vi "Get CSV Row.vi"(8 "error in (no error)":errorcluster, 11 "Trace in":refnum<class "Trace.lvclass">) -> (0 "error out":errorcluster, 2 "CSV Row":string, 3 "Trace out":refnum<class "Trace.lvclass">)   [LabVIEW 2014, in "Robot Actor Framework.lvlib" / "Trace.lvlib" / "Trace.lvclass"]
uses:
  Trace.lvclass
  Trace.lvclass/Trace.ctl
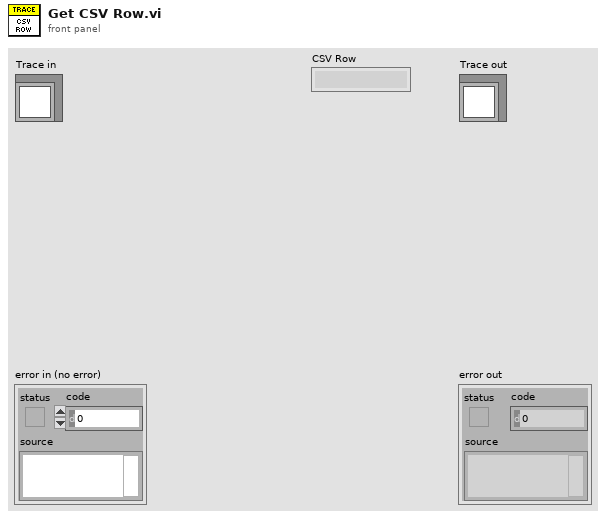
[diagram p1: front panel]
types:
  T1 = enum16{"Critical", "Error", "Warning", "Informational", "Debug"}
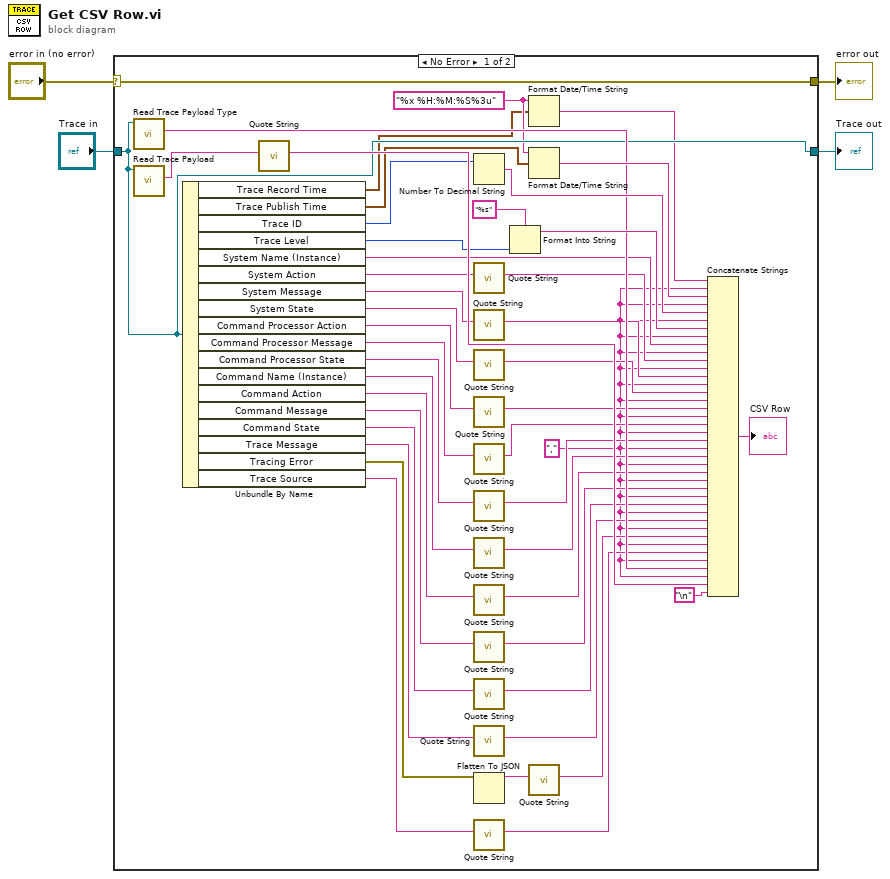
[diagram p0: block diagram]
diagram:
  n1 = case shown="No Error" "error in (no error)" {
    selector: "error in (no error)" -> [w50 w52]
    tunnel: [w50 w52] -> w3
    tunnel: [w33 w51] -> w1
    tunnel: "Trace in" -> [w33 w51]
    frame No Error {
      w8 = "%x %H:%M:%S%3u" ("time format string (%c)")
      w5 = "," ("string")
      n2 = call-dynamic "Read Trace Payload Type.vi"("Trace in"=w33) -> ("Trace Payload Type"=w41:string)  [unwired: 8 in, 2 out]
      n3 = call-dynamic "Read Trace Payload.vi"("Trace in"=w33) -> ("Trace Payload"=w44:string)  [unwired: 8 in, 2 out]
      n4 = Unbundle By Name(w33) -> ("Trace Record Time"=w7:timestamp, "Trace Publish Time"=w36:timestamp, "Trace ID"=w37:u32, "Trace Level"=w38:T1, "System Name (Instance)"=w39:string, "System Action"=w40:string, "System Message"=w20:string, "System State"=w32:string, "Command Processor Action"=w35:string, "Command Processor Message"=w18:string, "Command Processor State"=w29:string, "Command Name (Instance)"=w24:string, "Command Action"=w26:string, "Command Message"=w19:string, "Command State"=w22:string, "Trace Message"=w28:string, "Tracing Error"=w15:errorcluster, "Trace Source"=w12:string)
      n5 = call "Quote String.vi"("String In"=w44) -> ("Quoted String"=w43:string)  [unwired: 10 in]
      n6 = Number To Decimal String(number=w37) -> (decimal integer string=w49:string)  [unwired: 1 in]
      n7 = call "Quote String.vi"("String In"=w40) -> ("Quoted String"=w10:string)  [unwired: 10 in]
      n8 = call "Quote String.vi"("String In"=w20) -> ("Quoted String"=w9:string)  [unwired: 10 in]
      n9 = call "Quote String.vi"("String In"=w32) -> ("Quoted String"=w31:string)  [unwired: 10 in]
      n10 = call "Quote String.vi"("String In"=w35) -> ("Quoted String"=w34:string)  [unwired: 10 in]
      n11 = call "Quote String.vi"("String In"=w18) -> ("Quoted String"=w17:string)  [unwired: 10 in]
      n12 = call "Quote String.vi"("String In"=w29) -> ("Quoted String"=w30:string)  [unwired: 10 in]
      n13 = call "Quote String.vi"("String In"=w24) -> ("Quoted String"=w23:string)  [unwired: 10 in]
      n14 = call "Quote String.vi"("String In"=w26) -> ("Quoted String"=w25:string)  [unwired: 10 in]
      n15 = call "Quote String.vi"("String In"=w19) -> ("Quoted String"=w16:string)  [unwired: 10 in]
      n16 = call "Quote String.vi"("String In"=w22) -> ("Quoted String"=w21:string)  [unwired: 10 in]
      n17 = call "Quote String.vi"("String In"=w28) -> ("Quoted String"=w27:string)  [unwired: 10 in]
      n18 = Flatten To JSON(anything=w15) -> (JSON string=w14:string)  [unwired: 2 in, 1 out]
      n19 = call "Quote String.vi"("String In"=w12) -> ("Quoted String"=w11:string)  [unwired: 10 in]
      n20 = Format Into String(format string="%s", w38) -> (resulting string=w47:string)  [unwired: 2 in, 1 out]
      n21 = Format Date/Time String(time format string (%c)=w8, seconds (now)=w7) -> (date/time string=w6:string)  [unwired: 1 in]
      n22 = Format Date/Time String(time format string (%c)=w8, seconds (now)=w36) -> (date/time string=w42:string)  [unwired: 1 in]
      n23 = call "Quote String.vi"("String In"=w14) -> ("Quoted String"=w13:string)  [unwired: 10 in]
      n24 = Concatenate Strings(w6, w5, w42, w5, w49, w5, w47, w5, w39, w5, w10, w5, w9, w5, w31, w5, w34, w5, w17, w5, w30, w5, w23, w5, w25, w5, w16, w5, w21, w5, w27, w5, w13, w5, w11, w5, w41, w5, w43, "\n") -> (→"CSV Row":string)
    }
    frame Error {
    }
  }
  "error out" <- w3
  "Trace out" <- w1
